vi "Read Pixels and Copy to Display Image.vi"(0 "fpga interface in":refnum<k20>, 5 "display channel number":i32, 7 "serial channel display parameters":T4[](array[typedef]) {"RAW parameters"."bayer parameters"."blue gain" format="%_4g"; "RAW parameters"."bayer parameters"."green gain" format="%_4g"; "RAW parameters"."bayer parameters"."red gain" format="%_4g"; "RAW parameters"."bayer parameters"."algorithm" items=["Bilinear", "VNG"]; "RAW parameters"."bayer parameters"."pattern" items=["GB", "GR", "BG", "RG"]}, 9 "image metadata":T2, 11 "error in (no error)":errorcluster) -> (4 "fpga interface out":refnum<k20>, 6 "display image":T1, 15 "error out":errorcluster)   [LabVIEW 2023, in "GettingStarted_Common_148X_Host.lvlib"]
uses:
  GettingStarted_Common_148X_Host.lvlib
  <instrlib>/FlexRIO/CSI-2/v2/Common/Types/LLP Data Type.ctl
  <instrlib>/FlexRIO/CSI-2/v2/Common/NI CSI-2 API Common v2.lvlib
  <vilib>/vision/Image Controls.llb/IMAQ Image.ctl
  Types/Serial Channel Display Parameters.ctl
  FPGA/Common/Types/Image Metadata.ctl
  FPGA/Common/GettingStarted_Common_148X_FPGA.lvlib
  Types/RAW Interpretation for Display.ctl
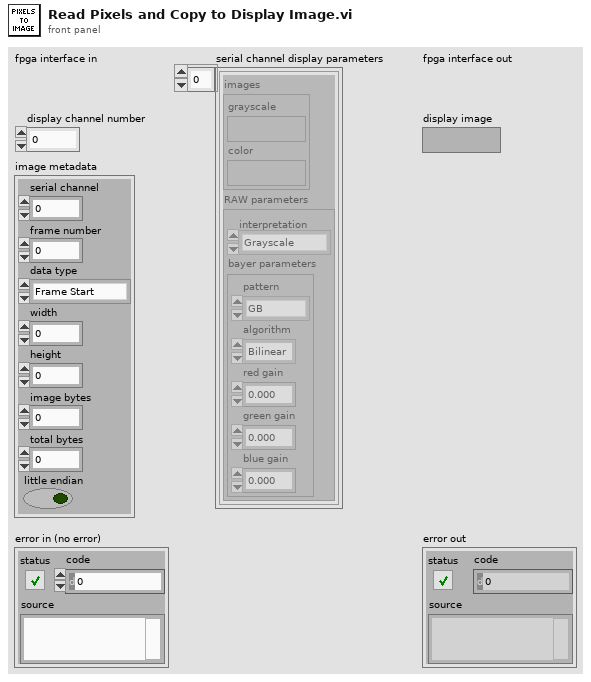
[diagram p1: front panel]
types:
  T1 = typedef "IMAQ Image.ctl" = refnum<image>
  T2 = typedef "GettingStarted_Common_148X_FPGA.lvlib/Image Metadata.ctl" = cluster{"serial channel":fxp<+,3,3>, "frame number":u16, "data type":T3, "width":u16, "height":u16, "image bytes":u32, "total bytes":u32, "little endian":bool}
  T3 = typedef "NI CSI-2 API Common v2.lvlib/LLP Data Type.ctl" = enum8{"Frame Start", "Frame End", "Line Start", "Line End", "End of Transmission", "Reserved 0", "Reserved 1", "Reserved 2", "Generic Short Packet 1", "Generic Short Packet 2", "Generic Short Packet 3", "Generic Short Packet 4", "Generic Short Packet 5", "Generic Short Packet 6", "Generic Short Packet 7", "Generic Short Packet 8", "Null", "Blanking Data", "Embedded 8-bit non Image Data", "Generic Long Packet 1", "Generic Long Packet 2", "Generic Long Packet 3", "Generic Long Packet 4", "Reserved 3", "YUV420 8-bit", "YUV420 10-bit", "Legacy YUV420 8-bit", "Reserved 4", "YUV420 8-bit Chroma Shifted", "YUV420 10-bit Chroma Shifted", "YUV422 8-bit", "YUV422 10-bit", "RGB444", "RGB555", "RGB565", "RGB666", "RGB888", "Reserved 5", "Reserved 6", "RAW 24", "RAW 6", "RAW 7", "RAW 8", "RAW 10", "RAW 12", "RAW 14", "RAW 16", "RAW 20", "User Defined 8-bit Data 1", "User Defined 8-bit Data 2", "User Defined 8-bit Data 3", "User Defined 8-bit Data 4", "User Defined 8-bit Data 5", "User Defined 8-bit Data 6", "User Defined 8-bit Data 7", "User Defined 8-bit Data 8", "USL Command", "Reserved 7", "Reserved 8", "Reserved 9", "Reserved 10", "Reserved 11", "Reserved 12", "LRTE EPD Spacer"}
  T4 = typedef "GettingStarted_Common_148X_Host.lvlib/Serial Channel Display Parameters.ctl" = cluster{"images":cluster{"grayscale":T1, "color":T1}, "RAW parameters":cluster{"interpretation":T5, "bayer parameters":cluster{"pattern":i32, "algorithm":i32, "red gain":dbl, "green gain":dbl, "blue gain":dbl}}}
  T5 = typedef "GettingStarted_Common_148X_Host.lvlib/RAW Interpretation for Display.ctl" = enum16{"Grayscale", "Bayer", "RGB", "YUV422", "YUV420", "Legacy YUV420"}
  T6 = cluster{"pattern":i32, "algorithm":i32, "red gain":dbl, "green gain":dbl, "blue gain":dbl}
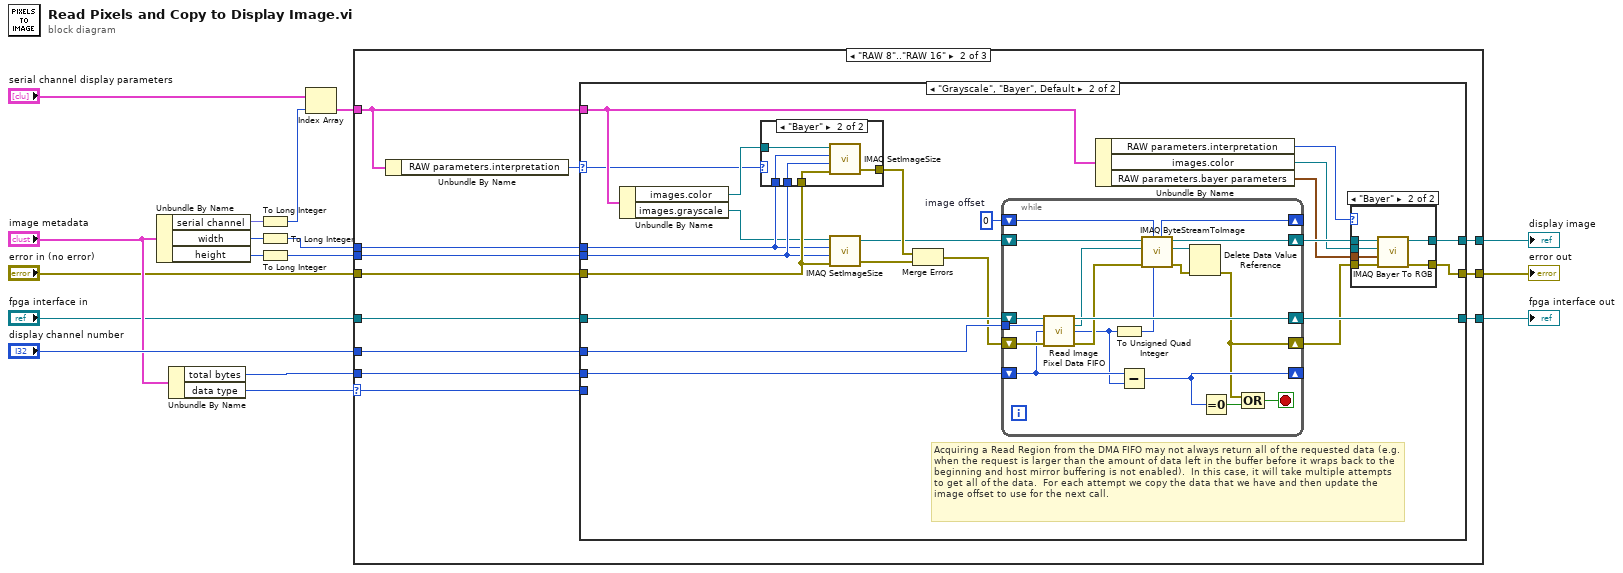
[diagram p0: block diagram]
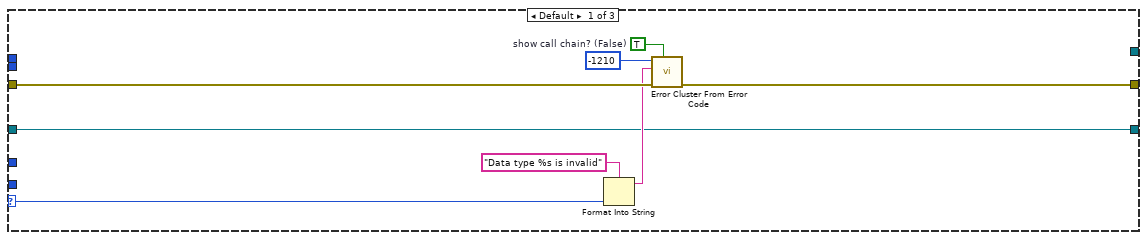
[diagram p2: hidden frame]
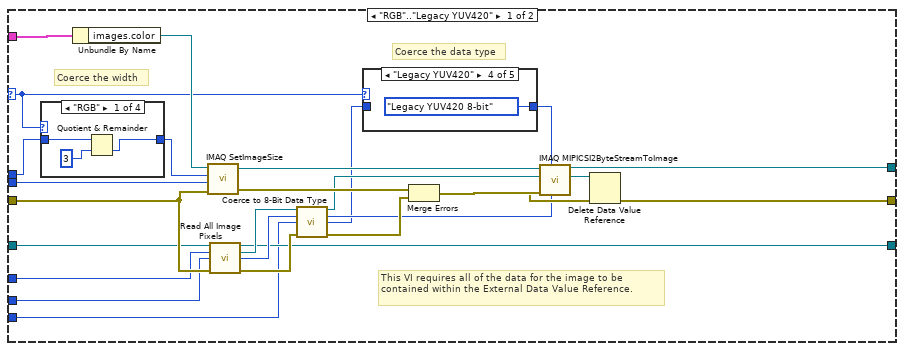
[diagram p3: hidden frame]
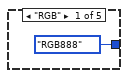
[diagram p4: hidden frame]
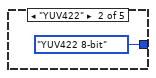
[diagram p5: hidden frame]
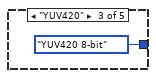
[diagram p6: hidden frame]
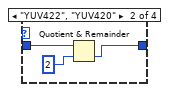
[diagram p8: hidden frame]
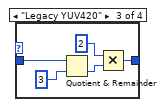
[diagram p9: hidden frame]
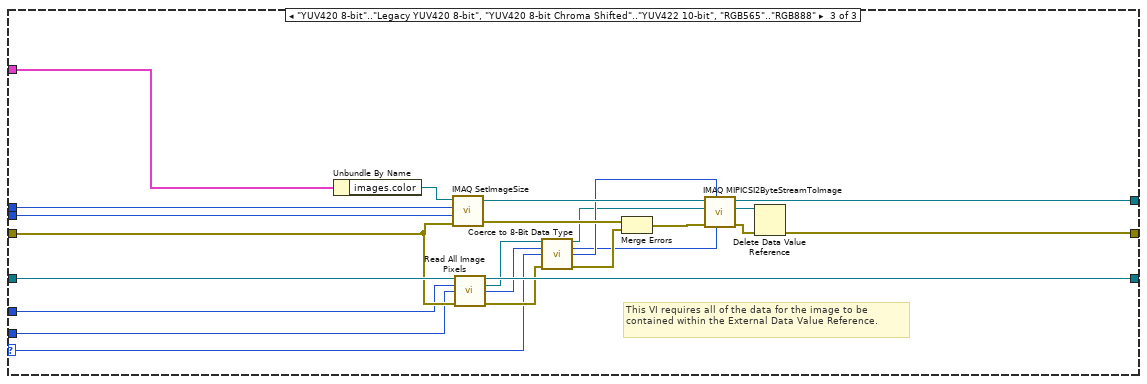
[diagram p13: hidden frame]
diagram:
  n1 = Unbundle By Name("image metadata") -> ("serial channel"=w13:fxp<+,3,3>, "width"=w9:u16, "height"=w10:u16)
  n2 = Unbundle By Name("image metadata") -> ("total bytes"=w16:u32, "data type"=w1:T3)
  n3 = To Long Integer(number=w13) -> (32bit integer=w11:i32)
  n4 = To Long Integer(number=w9) -> (32bit integer=w6:i32)
  n5 = To Long Integer(number=w10) -> (32bit integer=w7:i32)
  n6 = Index Array(array="serial channel display parameters", index=w11) -> (element=w3:T4)
  n7 = case shown="\"RAW 8\"..\"RAW 16\"" w1 {
    selector: w1 -> [w19 w26 w141]
    tunnel: w16 -> [_ w37 w151]
    tunnel: [w18 w36 w153] -> w15
    tunnel: "display channel number" -> [_ w35 w150]
    tunnel: "error in (no error)" -> [w23 w34 w154]
    tunnel: w7 -> [_ w33 w161]
    tunnel: w6 -> [_ w32 w160]
    tunnel: [_ w31 w149] -> w5
    tunnel: [w22 w30 w146] -> w4
    tunnel: w3 -> [_ w28 w158]
    tunnel: "fpga interface in" -> [w18 w29 w157]
    frame Default {
      w24 = TRUE  # show call chain? (False)
      n8 = Format Into String(format string="Data type %s is invalid" ("error message (\"\")"), w19) -> (resulting string=w20:string)  [unwired: 2 in, 1 out]
      n9 = call <vilib>:"Error Cluster From Error Code.vi"("show call chain? (False)"=w24, "error in (no error)"=w23, "error message (\"\")"=w20, "error code (0)"=-1210) -> ("error out"=w22:errorcluster)  [unwired: 5 in]
    }
    frame "RAW 8".."RAW 16" {
      n10 = Unbundle By Name(w28) -> ("RAW parameters.interpretation"=w27:T5)
      n11 = case shown="\"Grayscale\", \"Bayer\", Default" w27 {
        selector: w27 -> [w40 w82]
        tunnel: w37 -> [w47 w104]
        tunnel: [w51 w102] -> w36
        tunnel: w35 -> [w46 w101]
        tunnel: w34 -> [w52 w100]
        tunnel: w33 -> [w43 w98]
        tunnel: w32 -> [w42 w97]
        tunnel: [w49 w94] -> w31
        tunnel: [w50 w92] -> w30
        tunnel: w28 -> [w45 w87]
        tunnel: w29 -> [w48 w86]
        tunnel: w26 -> [w44 _]
        frame "RGB".."Legacy YUV420" {
          # "Coerce the data type"
          # "Coerce the width"
          # "This VI requires all of the data for the image to be contained within the External Data Value Reference."
          n12 = case shown="\"RGB\"" w40 {
            tunnel: w42 -> [w71 w74 w80 w81]
            tunnel: [w70 w73 w77 w81] -> w41
            frame "RGB" {
              n13 = Quotient & Remainder(x=w71, y=3) -> (floor(x/y)=w70:i32)  [unwired: 1 out]
            }
            frame "YUV422", "YUV420" {
              n14 = Quotient & Remainder(x=w74, y=2) -> (floor(x/y)=w73:i32)  [unwired: 1 out]
            }
            frame "Legacy YUV420" {
              n15 = Quotient & Remainder(x=w80, y=3) -> (floor(x/y)=w78:i32)  [unwired: 1 out]
              n16 = Multiply(x=2, y=w78) -> (x*y=w77:i32)
            }
            frame Default {
            }
          }
          n17 = Unbundle By Name(w45) -> ("images.color"=w64:T1)
          n18 = call "IMAQ SetImageSize"("error in (no error)"=w52, "Y Resolution"=w43, "X Resolution"=w41, "Image"=w64) -> ("error out"=w62:errorcluster, "Image Out"=w63:T1)  [unwired: 1 in]
          n19 = call "Read All Image Pixels.vi"("fpga inteface in"=w48, "display channel number"=w46, "image bytes"=w47, "error in (no error)"=w52) -> ("fpga interface out"=w51:refnum<k20>, "image pixel data region"=w57:refnum<data-value>, "elements in region"=w56:u32, "error out"=w58:errorcluster)  [unwired: 8 in]
          n20 = call "Coerce to 8-Bit Data Type.vi"("image pixel data region in"=w57, "image bytes in"=w56, "data type in"=w44, "error in (no error)"=w58) -> ("image pixel data region out"=w53:refnum<data-value>, "image bytes out"=w54:u32, "data type out"=w38:T3, "error out"=w55:errorcluster)  [unwired: 8 in]
          n21 = case shown="\"Legacy YUV420\"" w40 {
            tunnel: w38 -> [_ _ _ _ w69]
            tunnel: [LLP_Data_Type."RGB888" ("data type") LLP_Data_Type."YUV422 8-bit" ("data type") LLP_Data_Type."YUV420 8-bit" ("data type") LLP_Data_Type."Legacy YUV420 8-bit" ("data type") w69] -> w39
            frame "RGB" {
            }
            frame "YUV422" {
            }
            frame "YUV420" {
            }
            frame "Legacy YUV420" {
            }
            frame Default {
            }
          }
          n22 = Merge Errors(w62, w55) -> (w61:errorcluster)
          n23 = call "IMAQ MIPICSI2ByteStreamToImage"("Bytes to Copy"=w54, "Format"=w39, "error in (no error)"=w61, "Byte Stream In"=w53, "Image In"=w63) -> ("error out"=w60:errorcluster, "Byte Stream Out"=w59:refnum<data-value>, "Image Out"=w49:T1)  [unwired: 3 in, 1 out]
          n24 = Delete Data Value Reference(data value reference=w59, error in=w60) -> (error out=w50:errorcluster)  [unwired: 1 out]
        }
        frame "Grayscale", "Bayer", Default {
          w83 = u32 0  # image offset
          # "Acquiring a Read Region from the DMA FIFO may not always return all of the requested data (e.g. when the request is larger than the amount of data left in the buffer before it wraps back to the beginning and host mirror buffering is not enabled).  In this case, it will take multiple attempts to get all of the data.  For each attempt we copy the data that we have and then update the image offset to use for the next call."
          n25 = Unbundle By Name(w87) -> ("images.color"=w96:T1, "images.grayscale"=w91:T1)
          n26 = case shown="\"Bayer\"" w82 {
            tunnel: w100 -> [w105 w110]
            tunnel: [w105 w109] -> w99
            tunnel: w96 -> [_ w108]
            tunnel: w98 -> [_ w107]
            tunnel: w97 -> [_ w106]
            frame "Grayscale", Default {
            }
            frame "Bayer" {
              n27 = call "IMAQ SetImageSize"("error in (no error)"=w110, "Y Resolution"=w107, "X Resolution"=w106, "Image"=w108) -> ("error out"=w109:errorcluster)  [unwired: 1 in, 1 out]
            }
          }
          n28 = call "IMAQ SetImageSize"("error in (no error)"=w100, "Y Resolution"=w98, "X Resolution"=w97, "Image"=w91) -> ("error out"=w103:errorcluster, "Image Out"=w85:T1)  [unwired: 1 in]
          n29 = Merge Errors(w99, w103) -> (w84:errorcluster)
          n30 = while {
            tunnel: w101 -> [w127]
            shift-right: [w128] -> w102
            shift-left: w86 -> [w129]
            shift-right: [w113] -> w93
            shift-left: w84 -> [w126]
            shift-right: [w124] -> w95
            shift-left: w85 -> [w125]
            shift-right: [w116] -> _
            shift-left: w104 -> [w118]
            shift-right: [w112] -> _
            shift-left: w83 -> [w111]
            stop <- w114 stop-if-true
            n31 = call "Read Image Pixel Data FIFO.vi"("fpga inteface in"=w129, "display channel number"=w127, "number of elements"=w118, "error in (no error)"=w126) -> ("fpga interface out"=w128:refnum<k20>, "image pixel data region"=w123:refnum<data-value>, "elements in region"=w117:u32, "error out"=w122:errorcluster)  [unwired: 7 in, 1 out]
            n32 = To Unsigned Quad Integer(1:w117) -> (0:w121:u64)
            n33 = Subtract(x=w118, y=w117) -> (x-y=w116:u32)
            n34 = call "IMAQ ByteStreamToImage"("Bytes to Copy"=w121, "Image Byte Offset In"=w111, "error in (no error)"=w122, "Byte Stream In"=w123, "Image In"=w125) -> ("error out"=w119:errorcluster, "Byte Stream Out"=w120:refnum<data-value>, "Image Out"=w124:T1, "Image Byte Offset Out"=w112:u32)  [unwired: 2 in, 1 out]
            n35 = Delete Data Value Reference(data value reference=w120, error in=w119) -> (error out=w113:errorcluster)  [unwired: 1 out]
            n36 = Equal To 0?(x=w116) -> (x = 0?=w115:bool)
            n37 = Compound Arithmetic op=OR(w113, w115) -> (w114:bool)
          }
          n38 = Unbundle By Name(w87) -> ("RAW parameters.interpretation"=w88:T5, "images.color"=w89:T1, "RAW parameters.bayer parameters"=w90:T6)
          n39 = case shown="\"Bayer\"" w88 {
            tunnel: w95 -> [w130 w137]
            tunnel: [w130 w136] -> w94
            tunnel: w93 -> [w131 w135]
            tunnel: [w131 w134] -> w92
            tunnel: w89 -> [_ w133]
            tunnel: w90 -> [_ w132]
            frame "Grayscale", Default {
            }
            frame "Bayer" {
              n40 = call "IMAQ Bayer To RGB"("error in (no error)"=w135, "Bayer Parameters"=w132, "Image Dst"=w133, "Image Src"=w137) -> ("error out"=w134:errorcluster, "Image Dst Out"=w136:T1)  [unwired: 6 in]
            }
          }
        }
      }
    }
    frame "YUV420 8-bit".."Legacy YUV420 8-bit", "YUV420 8-bit Chroma Shifted".."YUV422 10-bit", "RGB565".."RGB888" {
      # "This VI requires all of the data for the image to be contained within the External Data Value Reference."
      n41 = Unbundle By Name(w158) -> ("images.color"=w159:T1)
      n42 = call "IMAQ SetImageSize"("error in (no error)"=w154, "Y Resolution"=w161, "X Resolution"=w160, "Image"=w159) -> ("error out"=w155:errorcluster, "Image Out"=w156:T1)  [unwired: 1 in]
      n43 = call "Read All Image Pixels.vi"("fpga inteface in"=w157, "display channel number"=w150, "image bytes"=w151, "error in (no error)"=w154) -> ("fpga interface out"=w153:refnum<k20>, "image pixel data region"=w144:refnum<data-value>, "elements in region"=w143:u32, "error out"=w145:errorcluster)  [unwired: 8 in]
      n44 = call "Coerce to 8-Bit Data Type.vi"("image pixel data region in"=w144, "image bytes in"=w143, "data type in"=w141, "error in (no error)"=w145) -> ("image pixel data region out"=w138:refnum<data-value>, "image bytes out"=w139:u32, "data type out"=w140:T3, "error out"=w142:errorcluster)  [unwired: 8 in]
      n45 = Merge Errors(w155, w142) -> (w152:errorcluster)
      n46 = call "IMAQ MIPICSI2ByteStreamToImage"("Bytes to Copy"=w139, "Format"=w140, "error in (no error)"=w152, "Byte Stream In"=w138, "Image In"=w156) -> ("error out"=w148:errorcluster, "Byte Stream Out"=w147:refnum<data-value>, "Image Out"=w149:T1)  [unwired: 3 in, 1 out]
      n47 = Delete Data Value Reference(data value reference=w147, error in=w148) -> (error out=w146:errorcluster)  [unwired: 1 out]
    }
  }
  "display image" <- w5
  "fpga interface out" <- w15
  "error out" <- w4
